vi "运维调试_采配水.vi"() -> ()   [LabVIEW 2016, in "PLC.lvlib"]
uses:
  PLC.lvlib
  <vilib>/Plasmionique/MB Master/MB_Master/MB_Master.lvclass
  <vilib>/Utility/miscctls.llb/LVPointTypeDef.ctl
  <vilib>/Plasmionique/MB Master/MB_Master_Serial/MB_Master_Serial.lvclass
  C:/Program Files (x86)/National Instruments/LabVIEW 2016/vi.lib/Plasmionique/MB Master/MB_Master/MB_Master.lvclass
  <vilib>/Instr/_visa.llb/VISA Configure Serial Port (Instr).vi
  <vilib>/Plasmionique/MB Master/MB Master.lvlib
panel:
  out "R118":i16 caption="多参数沉淀时间"
  in  "看门狗启用":bool
  out "R117":i16 caption="看门狗设置值"
  out "R33":i16 caption="看门狗计时器"
  in  "下载模式":bool
  in  "R116":i16(ring) caption="储水水体选择" items=["自来水", "采水泵"]
  out "当前启动泵号":u16(ring) items=["1号水样泵", "2号水样泵"]
  out "R113":i16 caption="储水时间设定"
  out "R25":i16
  in  "V14NC":bool
  out "R24":i16
  in  "V14NO":bool
  out "X2":bool caption="X1"
  out "采配水版本号":string
  out "R23":i16 caption="清洗频次计数"
  out "R112":i16 caption="清洗频次设定"
  out "R22":i16
  in  "V13NC":bool
  out "R111":i16 caption="排液时间"
  out "通讯故障":bool
  out "R21":i16
  in  "V13NO":bool
  out "R20":i16
  in  "M1-2":bool
  in  "潜水泵工作模式":u16(ring) items=["泵1单泵单管路", "泵2单泵单管路", "潜水泵双泵双管路", "自吸泵双泵双管路"]
  out "X11":bool caption="废液报警"
  out "X10":bool caption="自来水检测"
  out "X9":bool caption="泵2过载报警"
  out "X8":bool caption="泵1过载报警"
  out "X7":bool caption="断电检测"
  out "X6":bool caption="开门检测"
  out "X5":bool caption="烟雾检测"
  out "X4":bool caption="漏水检测"
  out "X3":bool caption="进样检测"
  out "X1":bool
  out "X0":bool caption="采样池液位开关"
  out "R109":i16 caption="配水时间"
  out "集成报警信息":string
  out "R108":i16 caption="自来水报警"
  out "R107":i16 caption="采水池液位报警设置"
  out "R106":i16 caption="进样超时设置"
  out "R105":i16 caption="二级清洗时间"
  out "R104":i16 caption="一级清洗时间"
  out "R103":i16 caption="外部管路清洗时间"
  out "R102":i16 caption="静置沉淀时间"
  out "R101":i16 caption="内部管路润洗时间"
  out "R100":i16 caption="外部管路润洗时间"
  out "R2":i16
  out "R1":i16
  out "多列列表框":i32(listbox)
  out "R19":i16
  in  "V6":bool
  out "R18":i16
  in  "V5":bool
  out "R17":i16
  in  "V4":bool
  out "R16":i16
  in  "V3":bool
  out "R15":i16
  in  "V2":bool
  out "R14":i16
  in  "M2":bool
  out "R13":i16
  in  "V1":bool
  out "R12":i16
  in  "M1-1":bool
  in  "返回":bool
  in  "参数设置":bool
  in  "单步启动":bool
  in  "启动":bool
  in  "停止":bool
  # "看门狗设置"
  # "S"
  # "S"
  # "S"
  # "S"
  # "次"
  # "次"
  # "S"
  # "S"
  # "S"
  # "S"
  # "S"
  # "S"
  # "S"
  # "S"
  # "S"
  # "S"
  # "S"
  # "单步计时："
  # "s"
  # "流程计时："
  # "s"
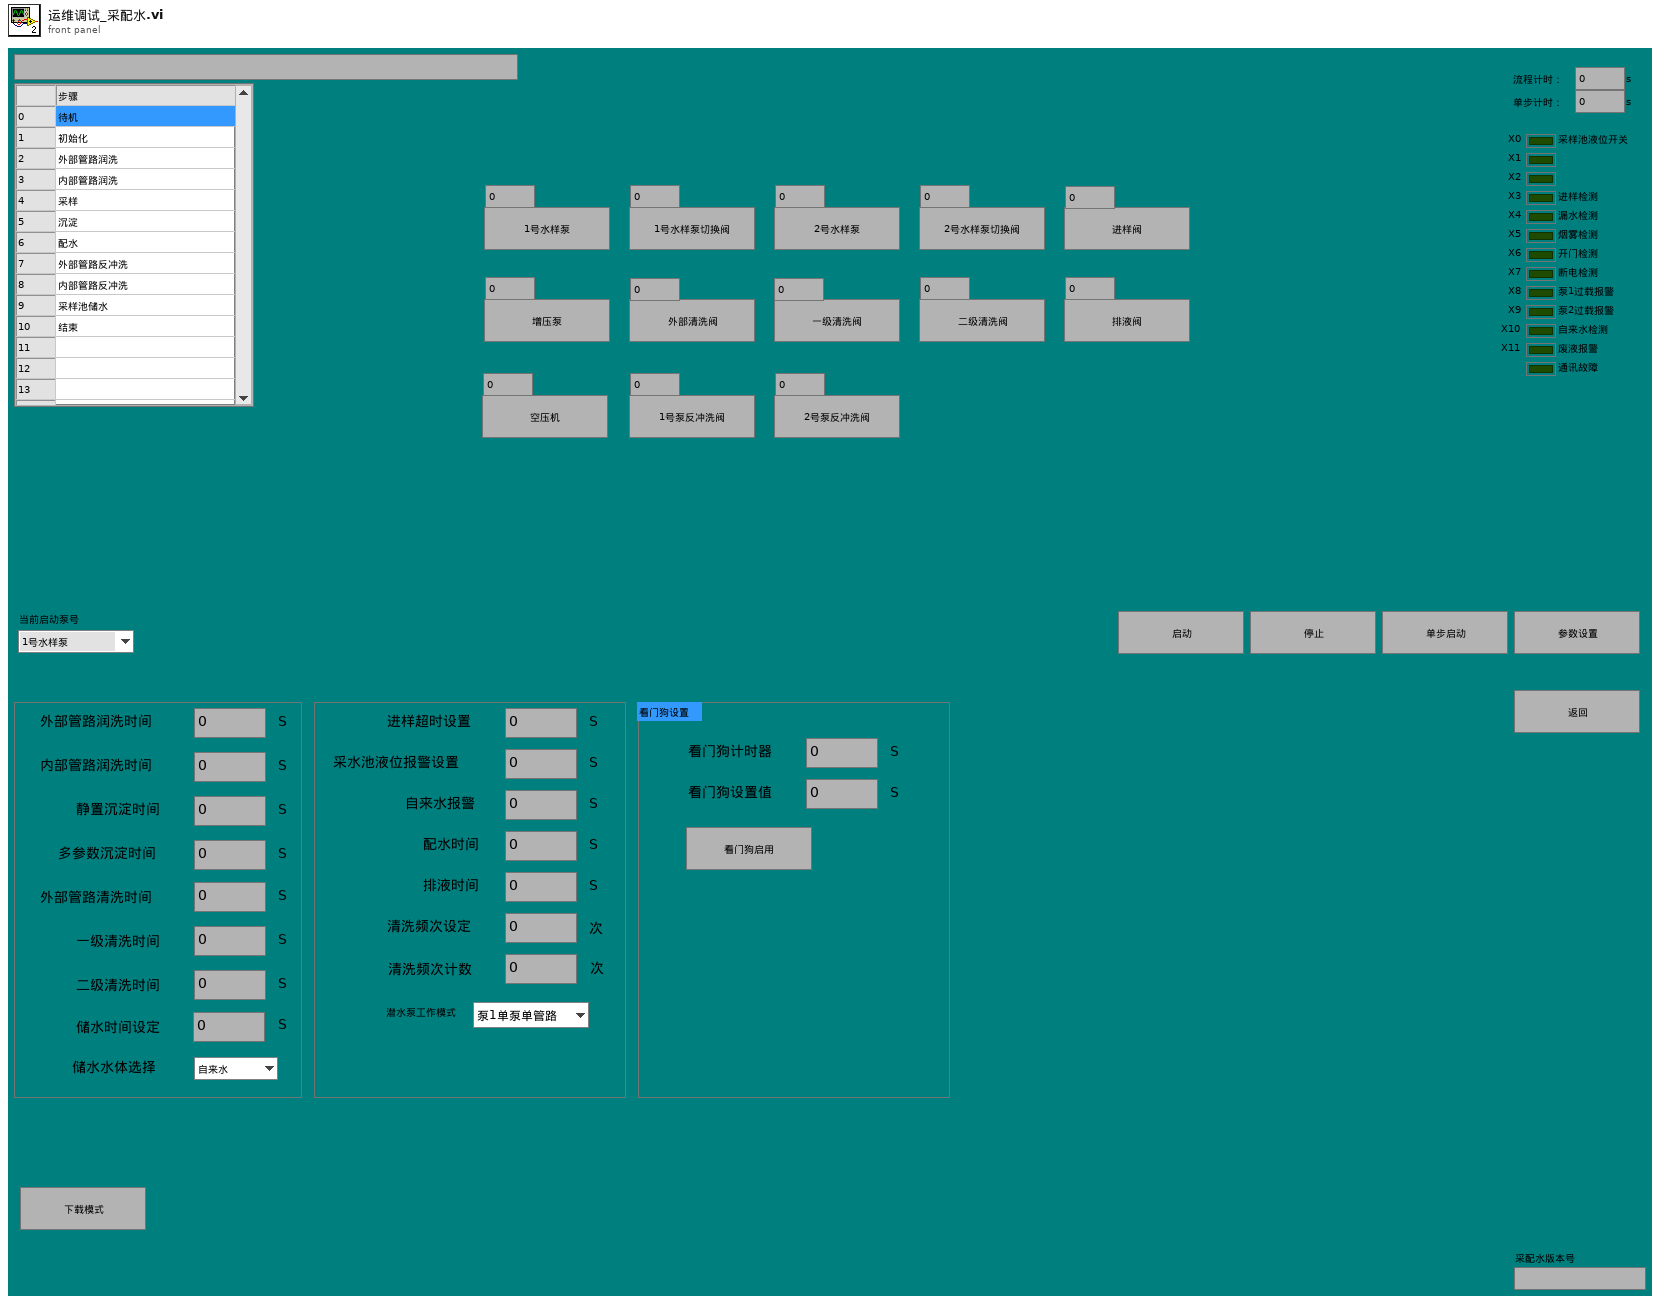
[diagram p1: front panel]
types:
  T1 = typedef "LVPointTypeDef.ctl" = cluster{"Horizontal":i16, "Vertical":i16}
  T2 = cluster{"命令":string, "数据":cluster{"starting address":u16, "holding register value":u16}}
  T3 = cluster{"时间标识":timestamp, "设备":string, "日志信息":string}
  T4 = cluster{"R0":i16, "R1":i16, "R2":i16, "R3":i16, "R4":i16, "R5":i16, "R6":i16, "R7":i16, "R8":i16, "R9":i16, "R10":i16, "R11":i16, "R12":i16, "R13":i16, "R14":i16, "R15":i16, "R16":i16, "R17":i16, "R18":i16, "R19":i16, "R20":i16, "R21":i16, "R22":i16, "R23":i16, "R24":i16, "R25":i16, "R26":i16, "R27":i16, "R28":i16, "R29":i16, "R30":i16, "R31":i16, "R32":i16, "R33":i16, "R34":i16}
  T5 = cluster{"R100":i16, "R101":i16, "R102":i16, "R103":i16, "R104":i16, "R105":i16, "R106":i16, "R107":i16, "R108":i16, "R109":i16, "R110":i16, "R111":i16, "R112":i16, "R113":i16, "R114":i16, "R115":i16, "R116":i16, "R117":i16, "R118":i16, "R119":i16}
  T6 = cluster{"seconds since 1Jan1904":timestamp, "table输入":string, string, "table输入":string}
  T7 = cluster{"时间标识":timestamp, "设备":string, "日志信息":string, "流程参数":string}
  T8 = cluster{"命令":string, cluster{"starting address":u16, "holding register value":u16}}
  T9 = cluster{"命令":string, "数据":cluster{"starting address":u16, "holding register values":u16[]}}
  T10 = cluster{"命令":string, "data":cluster{"starting address":u16, "coil values":bool[]}}
  T11 = cluster{"测试模式":enum16{"正常测试", "集成干预"}, "参数启用":cluster{"氨氮":bool, "总磷总氮":bool, "CODMn":bool, "CODcr":bool, "多参数":bool}}
  T12 = enum32{"Bad", "Idle", "Run top level", "Running"}
  T13 = cluster{"baud rate (bps)":u32, "stop bits":u16, "parity":u16, "flow control":u16, "timeout":u32, "retries":i32}
  T14 = cluster{"starting address":u16, "holding register values":u16[]}
  T15 = cluster{"starting address":u16, "holding register value":u16}
  T16 = cluster{"starting address":u16, "coil values":bool[]}
  T17 = cluster{"Registers[0]":u16, "Registers[1]":u16, "Registers[2]":u16, "Registers[3]":u16, "Registers[4]":u16, "Registers[5]":u16, "Registers[6]":u16, "Registers[7]":u16, "Registers[8]":u16, "Registers[9]":u16, "Registers[10]":u16, "Registers[11]":u16, "Registers[12]":u16, "Registers[13]":u16, "Registers[14]":u16, "Registers[15]":u16, "Registers[16]":u16, "Registers[17]":u16, "Registers[18]":u16, "Registers[19]":u16, "Registers[20]":u16, "Registers[21]":u16, "Registers[22]":u16, "Registers[23]":u16, "Registers[24]":u16, "Registers[25]":u16, "Registers[26]":u16, "Registers[27]":u16, "Registers[28]":u16, "Registers[29]":u16, "Registers[30]":u16, "Registers[31]":u16, "Registers[32]":u16, "Registers[33]":u16, "Registers[34]":u16}
  T18 = cluster{"数组 2[0]":sgl, "数组 2[1]":sgl, "数组 2[2]":sgl, "数组 2[3]":sgl, "数组 2[4]":sgl}
  T19 = cluster{"Registers[0]":u16, "Registers[1]":u16, "Registers[2]":u16, "Registers[3]":u16, "Registers[4]":u16, "Registers[5]":u16}
  T20 = cluster{"Registers[0]":u16, "Registers[1]":u16, "Registers[2]":u16, "Registers[3]":u16, "Registers[4]":u16, "Registers[5]":u16, "Registers[6]":u16, "Registers[7]":u16, "Registers[8]":u16, "Registers[9]":u16, "Registers[10]":u16, "Registers[11]":u16, "Registers[12]":u16, "Registers[13]":u16, "Registers[14]":u16, "Registers[15]":u16, "Registers[16]":u16, "Registers[17]":u16, "Registers[18]":u16, "Registers[19]":u16}
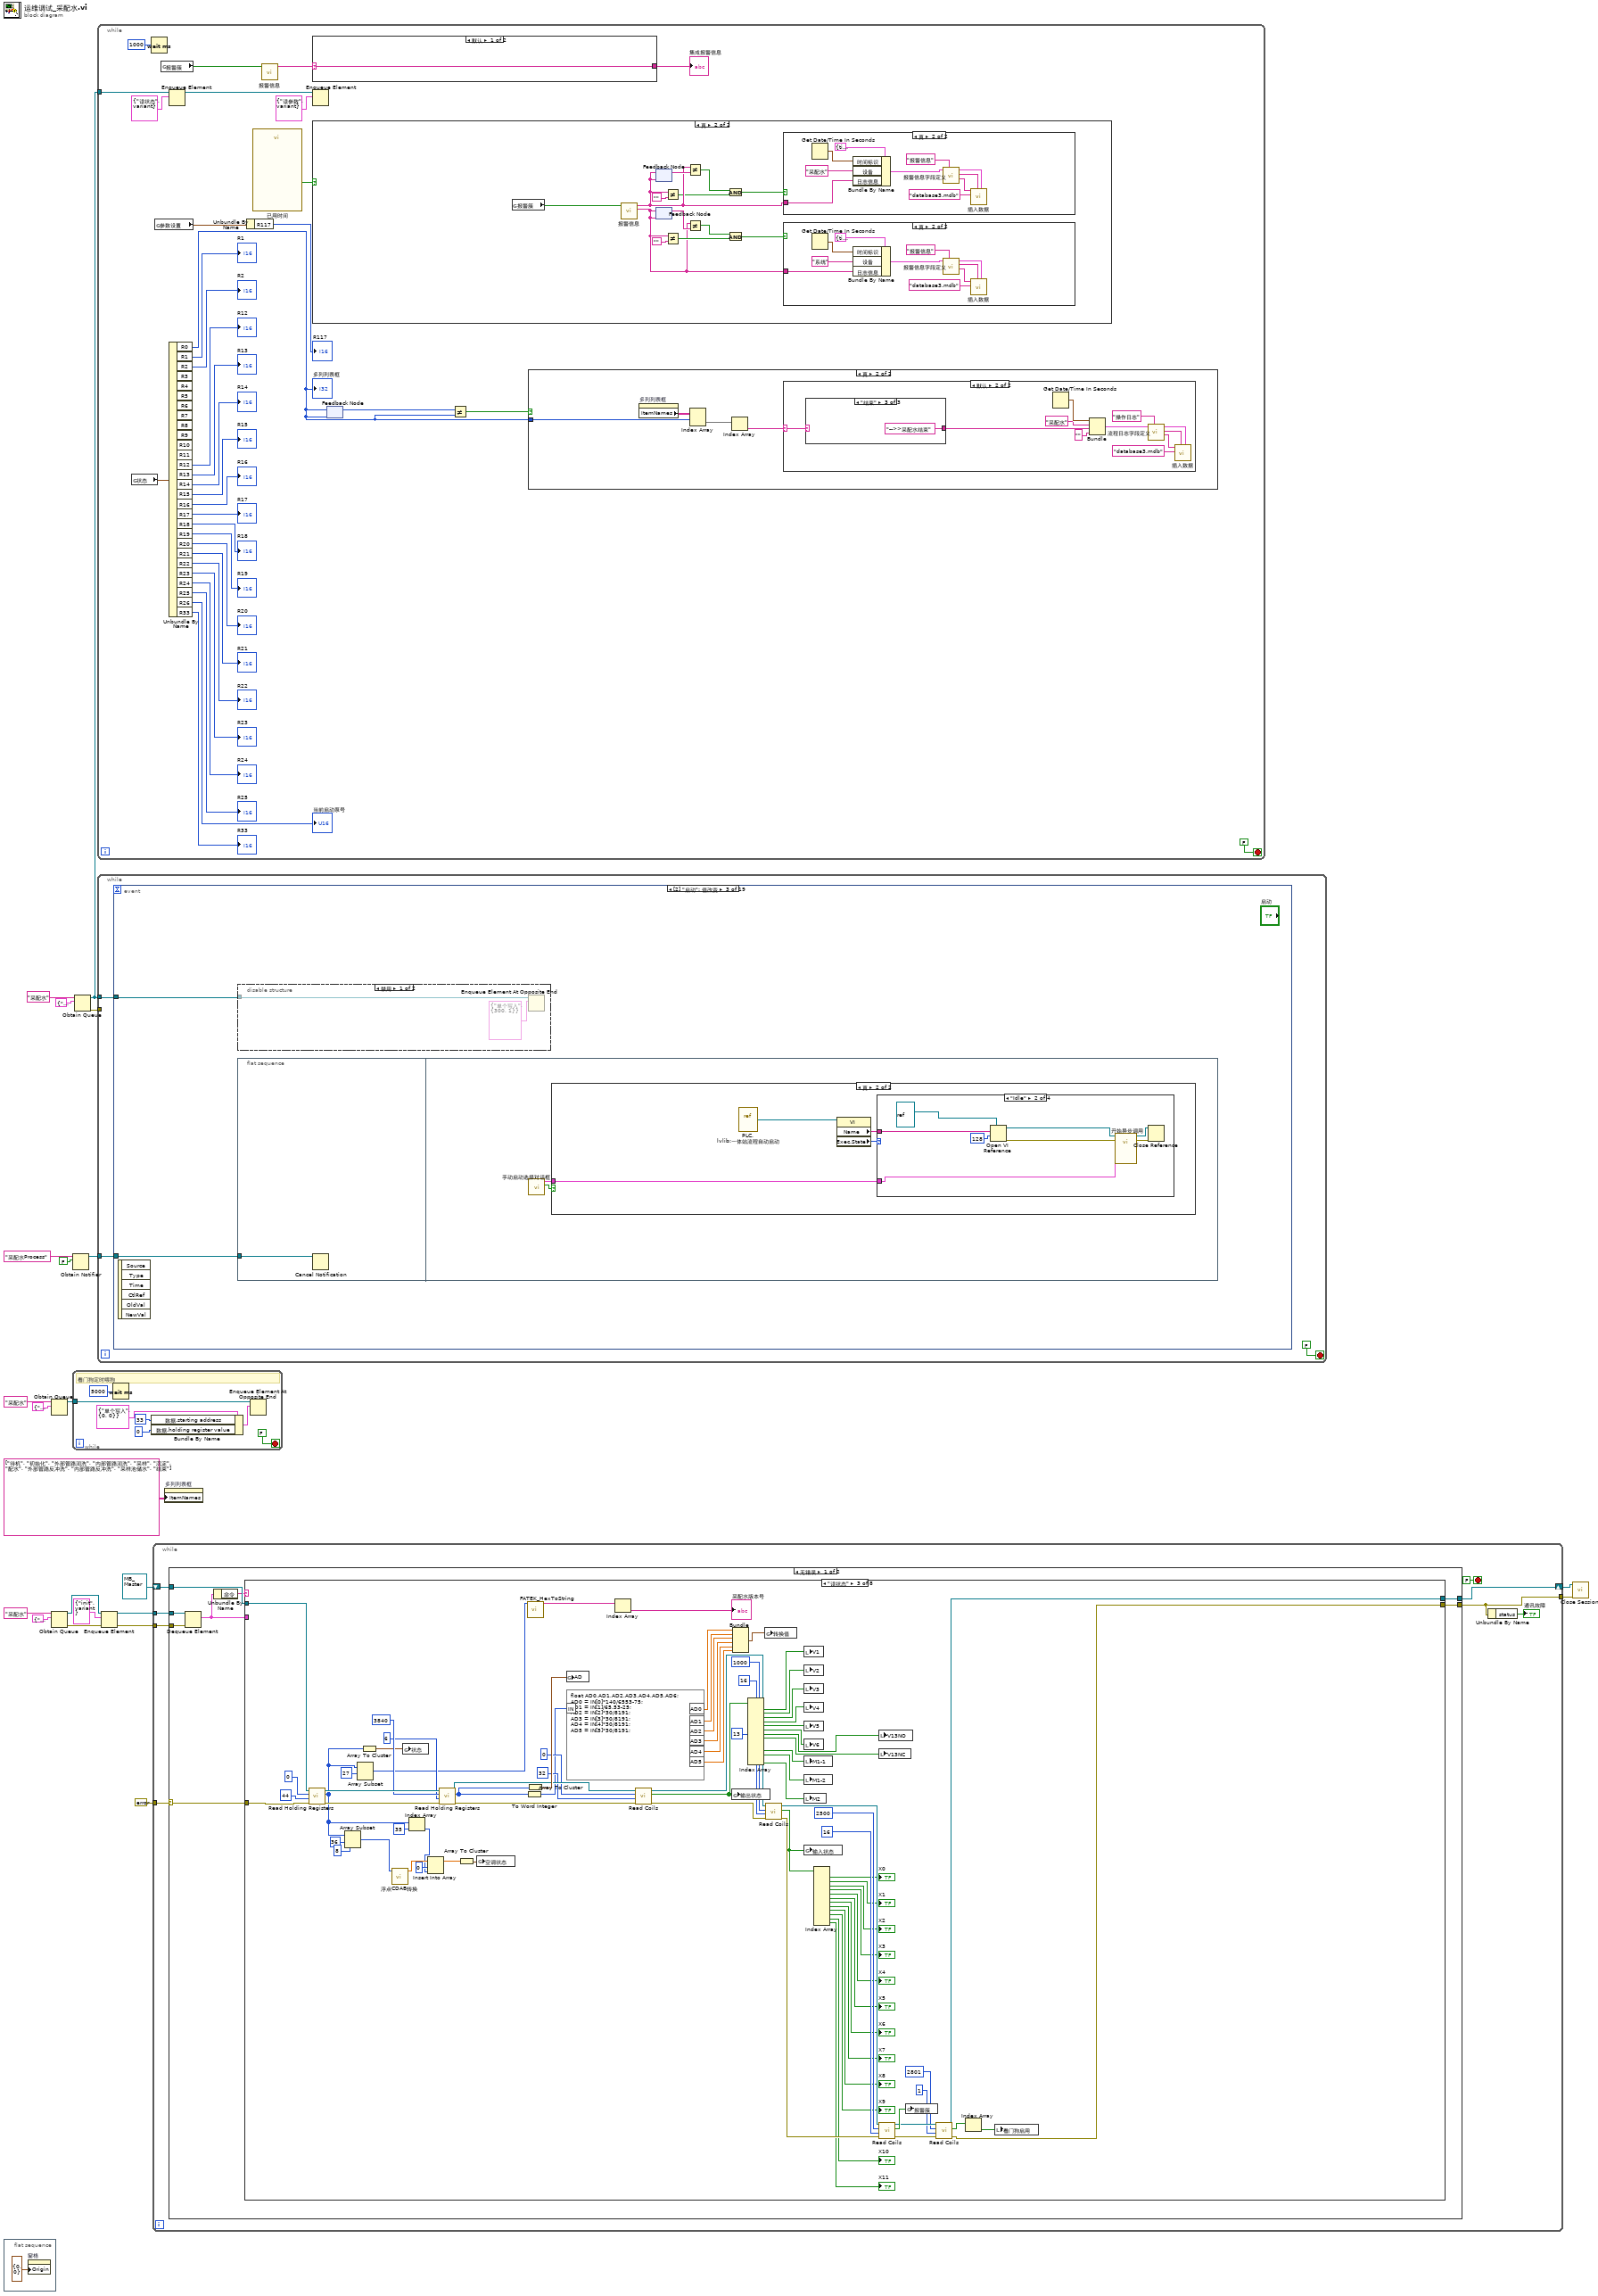
[diagram p0: block diagram]
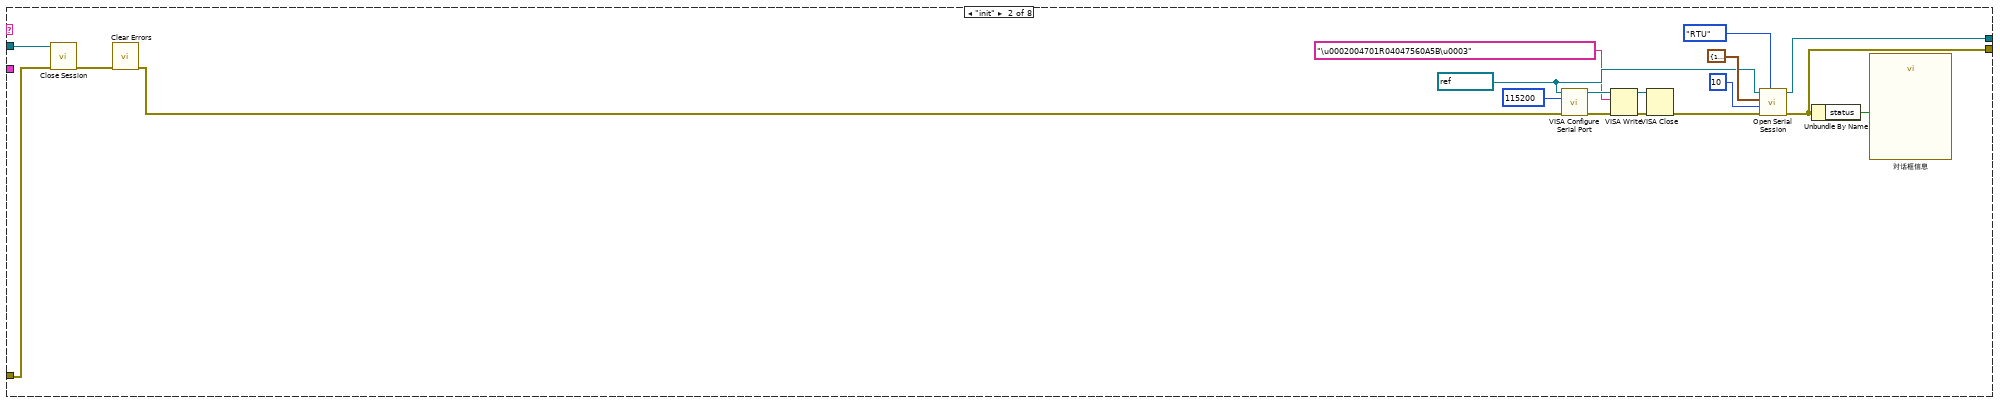
[diagram p3: hidden frame]
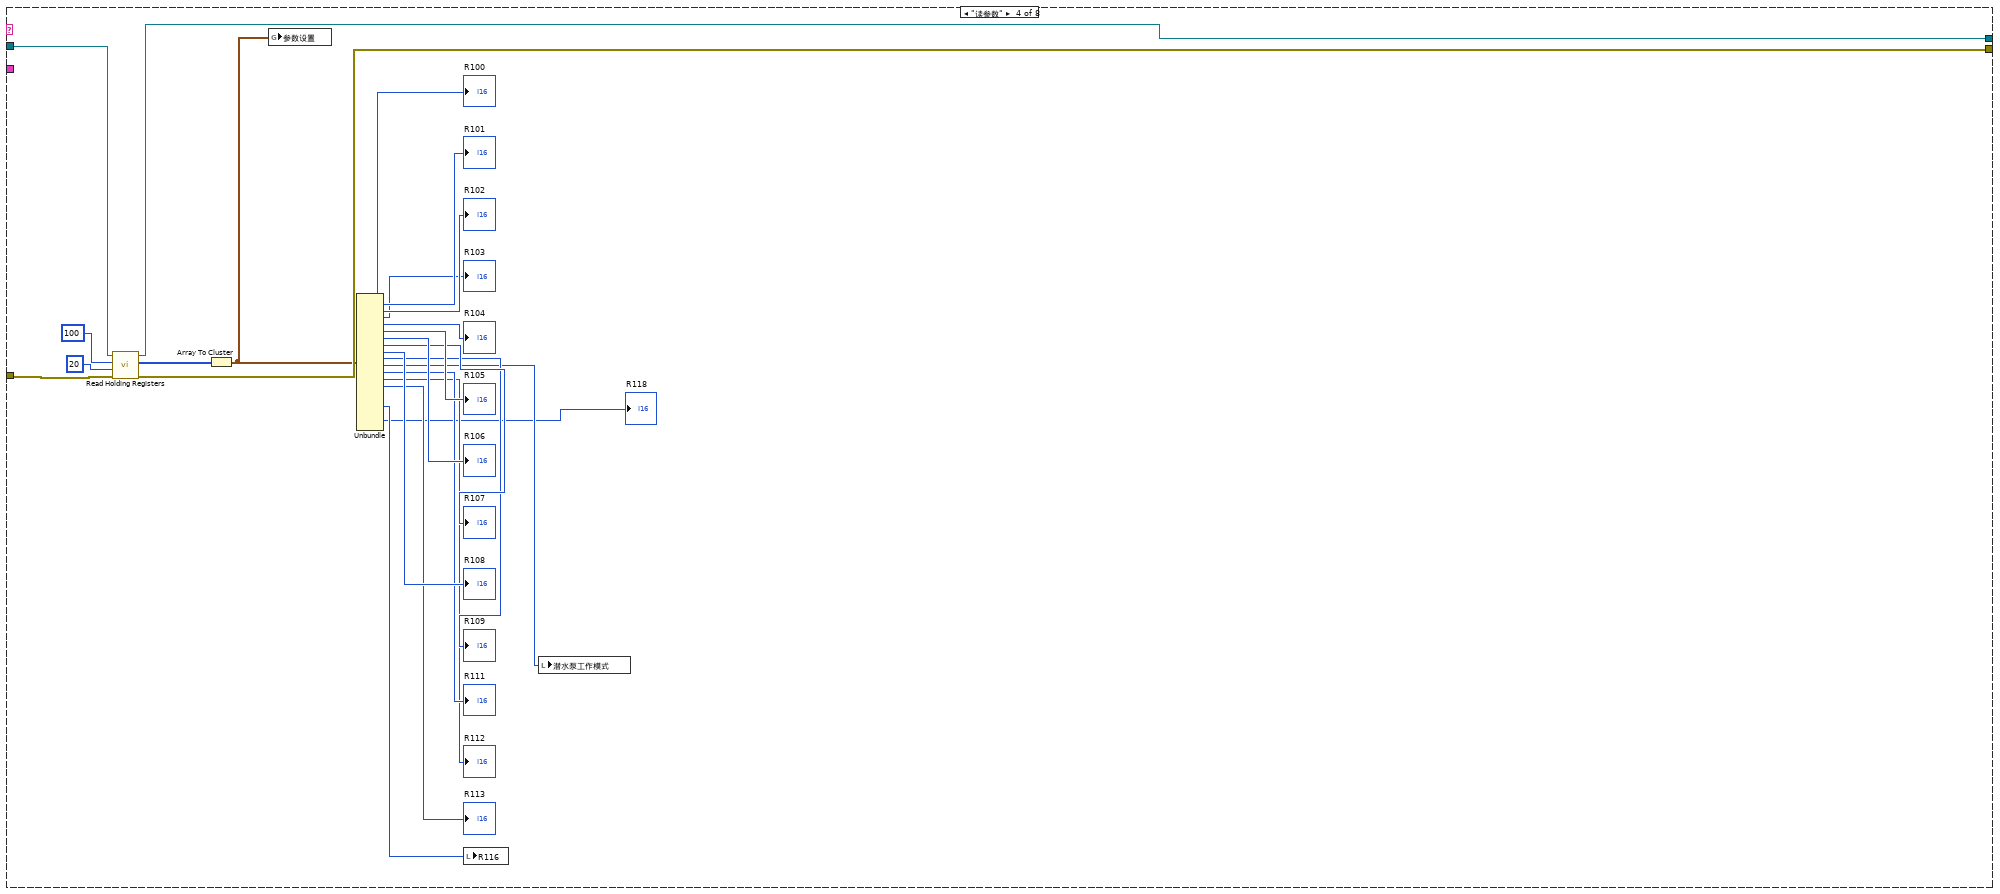
[diagram p4: hidden frame]
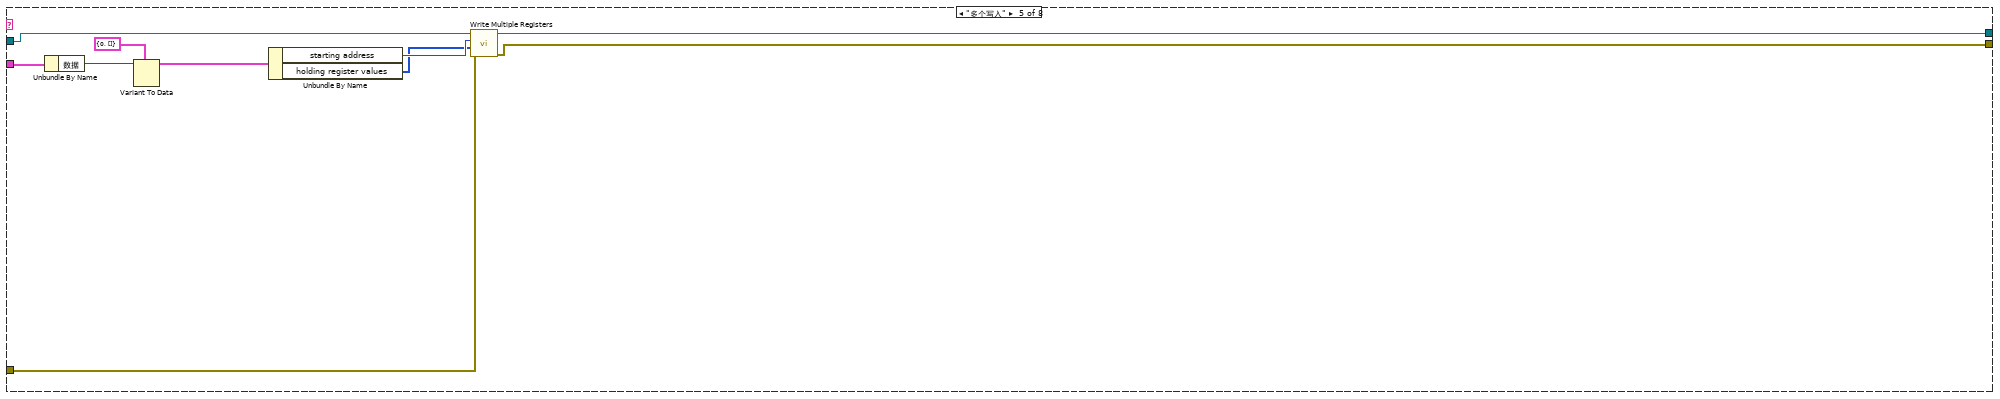
[diagram p5: hidden frame]
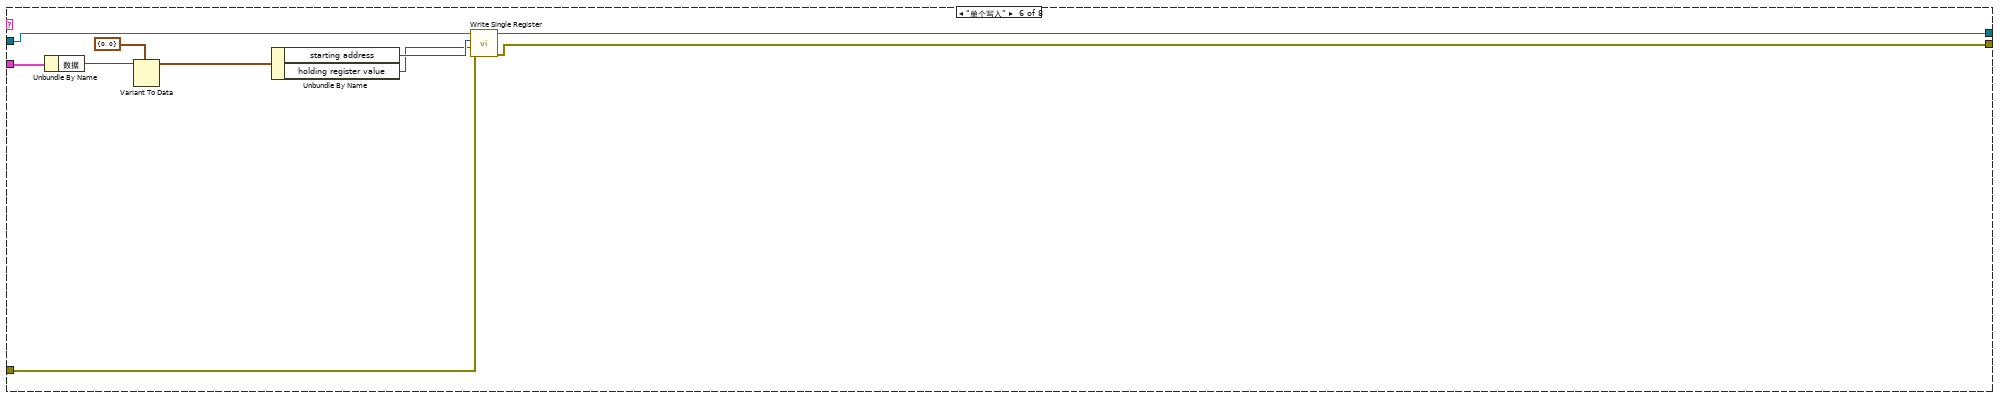
[diagram p6: hidden frame]
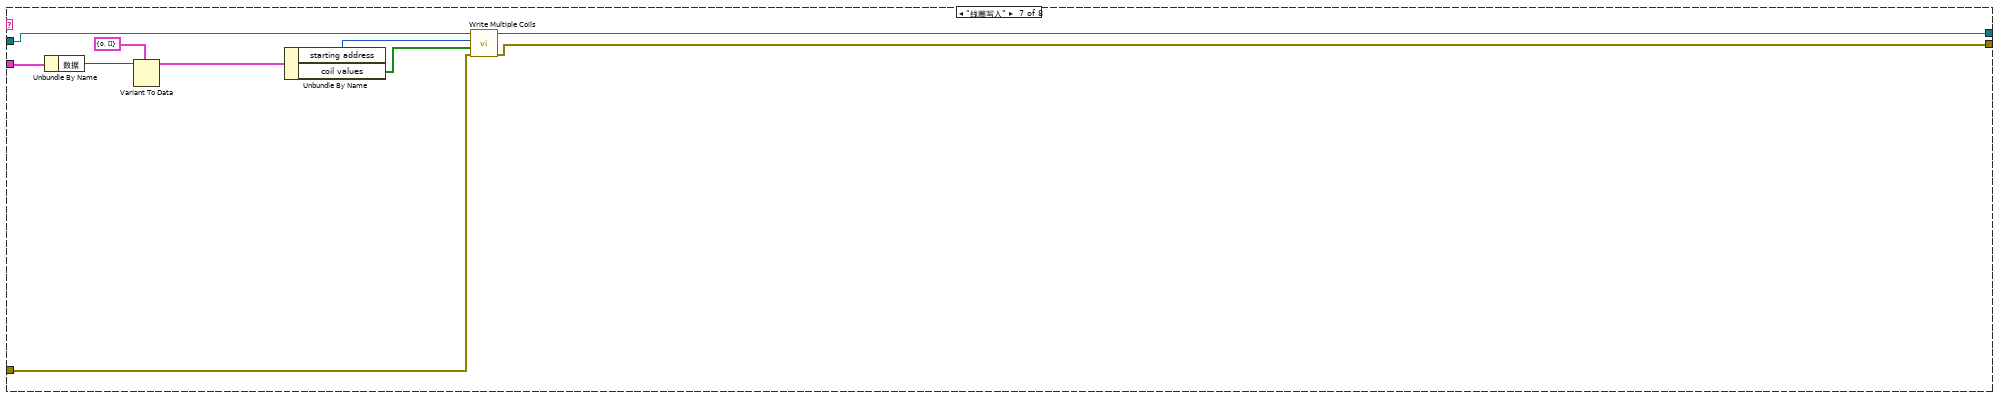
[diagram p7: hidden frame]
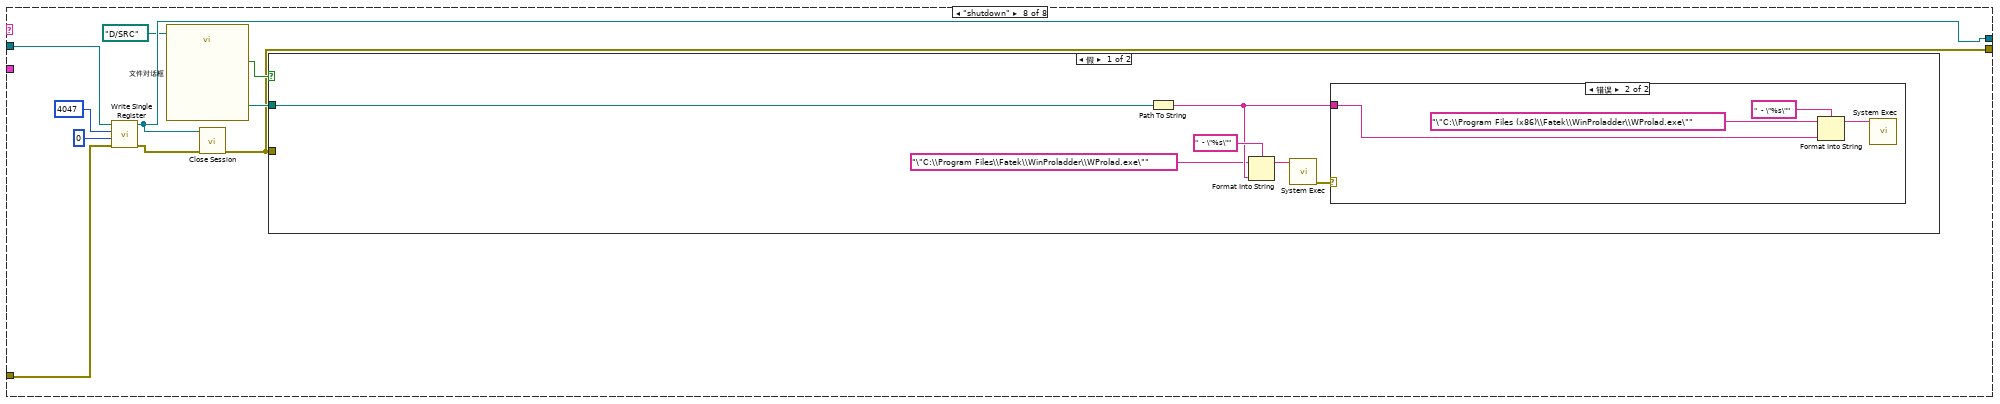
[diagram p8: hidden frame]
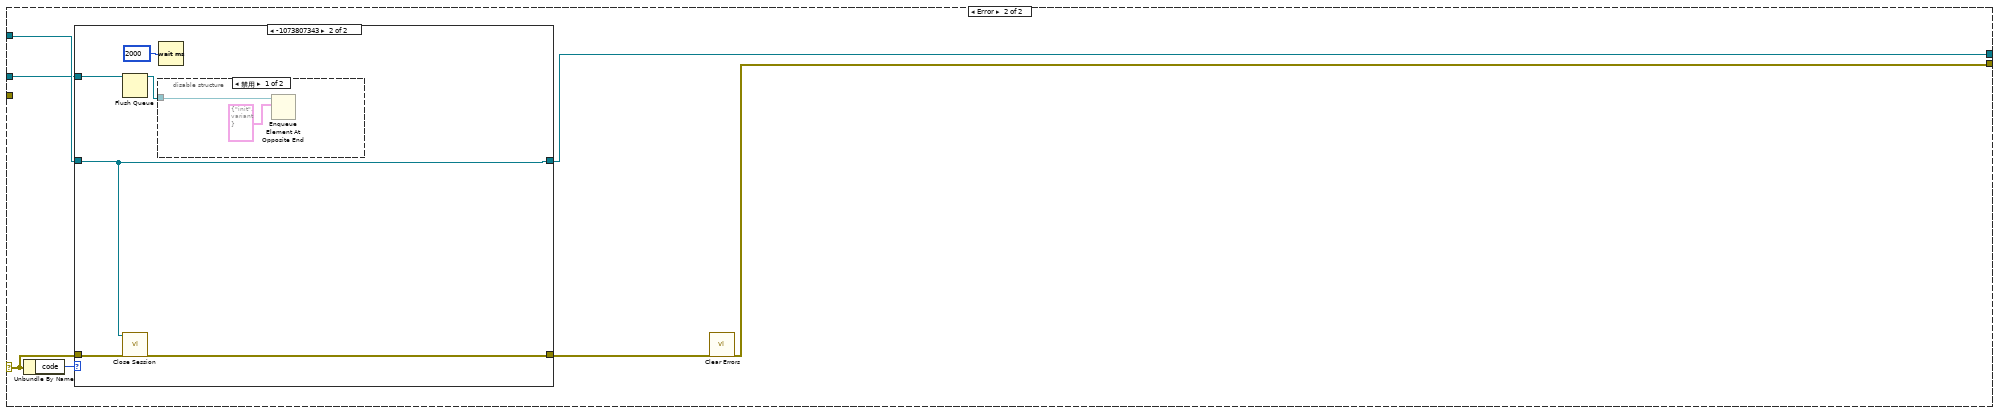
[diagram p11: hidden frame]
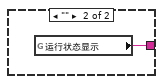
[diagram p17: hidden frame]
diagram:
  n1 = flat-sequence {
    frame #0 {
      n2 = property on="窗格" class="Pane"("Origin"=T1 {"Horizontal"=0, "Vertical"=0} ("原点")) -> ()  [unwired: 2 in, 2 out]
    }
  }
  n3 = Obtain Queue(name (unnamed)="采配水" ("名称（未命名）"), element data type=cluster{"命令":string, "数据":variant} {"命令"="", "数据"=variant}) -> (queue out=w1:refnum<queue>)  [unwired: 3 in, 2 out]
  n4 = Obtain Queue(name (unnamed)="采配水" ("名称（未命名）"), element data type=cluster{"命令":string, "数据":variant} {"命令"="", "数据"=variant}) -> (queue out=w12:refnum<queue>, error out=w11:errorcluster)  [unwired: 3 in, 1 out]
  n5 = Obtain Notifier(name (unnamed)="采配水Process" ("名称（未命名）"), notification data type=FALSE) -> (notifier out=w15:refnum<notifier>)  [unwired: 2 in, 2 out]
  n6 = while {
    tunnel: w1 -> [w26]
    stop <- FALSE stop-if-true
    # "看门狗定时喂狗"
    n7 = Wait (ms)(milliseconds to wait=u32 5000 ("等待时间（毫秒）")) -> ()  [unwired: 1 out]
    n8 = Bundle By Name(cluster=T2 {"命令"="单个写入", "数据"={"starting address"=0, "holding register value"=0}} ("元素"), "数据.starting address"=u16 33, "数据.holding register value"=u16 0) -> (w27:T2)
    n9 = Enqueue Element At Opposite End(queue=w26, element=w27) -> ()  [unwired: 2 in, 3 out]
  }
  n10 = Obtain Queue(name (unnamed)="采配水" ("名称（未命名）"), element data type=cluster{"命令":string, "数据":variant} {"命令"="", "数据"=variant}) -> (queue out=w19:refnum<queue>, error out=w20:errorcluster)  [unwired: 3 in, 1 out]
  n11 = while {
    tunnel: w19 -> [w63]
    stop <- FALSE stop-if-true
    n12 = global read "采配水全局变量.vi" "状态"() -> (w61:T4)
    n13 = Wait (ms)(milliseconds to wait=u32 1000 ("等待时间（毫秒）")) -> ()  [unwired: 1 out]
    n14 = global read "采配水全局变量.vi" "参数设置"() -> (w32:T5)
    n15 = global read "采配水全局变量.vi" "报警簇"() -> (w49:bool[])
    n16 = Enqueue Element(queue=w63, element=cluster{"命令":string, "数据":variant} {"命令"="读状态", "数据"=variant} ("元素")) -> (queue out=w44:refnum<queue>)  [unwired: 2 in, 2 out]
    n17 = Unbundle By Name(w61) -> ("R0"=w42:i16, "R1"=→"R1":i16, "R2"=→"R2":i16, "R12"=→"R12":i16, "R13"=→"R13":i16, "R14"=→"R14":i16, "R15"=→"R15":i16, "R16"=→"R16":i16, "R17"=→"R17":i16, "R18"=→"R18":i16, "R19"=→"R19":i16, "R20"=→"R20":i16, "R21"=→"R21":i16, "R22"=→"R22":i16, "R23"=→"R23":i16, "R24"=→"R24":i16, "R25"=→"R25":i16, "R26"=→"当前启动泵号":i16, "R33"=→"R33":i16)  [unwired: 9 out]
    "多列列表框" <- w42
    n18 = Unbundle By Name(w32) -> ("R117"=→"R117":i16)
    n19 = call "已用时间"() -> ("Time has Elapsed"=w47:bool)  [unwired: 12 in, 7 out]
    n20 = call "报警信息.vi"("报警簇"=w49) -> ("采配水报警信息"=w41:string)  [unwired: 9 in, 1 out]
    n21 = case shown="默认" w41 {
      selector: w41 -> [w98 _]
      tunnel: [w98 w99] -> w48
      frame Default {
      }
      frame "" {
        n22 = global read "采配水全局变量.vi" "运行状态显示"() -> (w99:string)
      }
    }
    "集成报警信息" <- w48
    n23 = Enqueue Element(queue=w44, element=cluster{"命令":string, "数据":variant} {"命令"="读参数", "数据"=variant} ("元素")) -> ()  [unwired: 2 in, 3 out]
    n24 = case shown="真" w47 {
      frame False {
      }
      frame True {
        n25 = global read "采配水全局变量.vi" "报警簇"() -> (w77:bool[])
        n26 = call "报警信息.vi"("报警簇"=w77) -> ("系统报警信息"=w66:string, "采配水报警信息"=w73:string)  [unwired: 9 in]
        n27 = feedback #1(w73) -> (w76:string)
        n28 = feedback-in #1(w73) -> ()
        n29 = feedback #2(w66) -> (w67:string)
        n30 = feedback-in #2(w66) -> ()
        n31 = Not Equal?(x=w73, y="") -> (x != y?=w71:bool)
        n32 = Not Equal?(x=w66, y="") -> (x != y?=w70:bool)
        n33 = Not Equal?(x=w73, y=w76) -> (x != y?=w75:bool)
        n34 = Not Equal?(x=w66, y=w67) -> (x != y?=w68:bool)
        n35 = And(x=w75, y=w71) -> (x .and. y?=w74:bool)
        n36 = And(x=w68, y=w70) -> (x .and. y?=w65:bool)
        n37 = case shown="真" w74 {
          tunnel: w73 -> [_ w88]
          frame False {
          }
          frame True {
            n38 = Get Date/Time In Seconds() -> (seconds since 1Jan1904=w90:timestamp)
            n39 = Bundle By Name(cluster=T3 {"时间标识"=timestamp(0 s since 1904-01-01), "设备"="", "日志信息"=""} ("data in"), "时间标识"=w90, "设备"="采配水", "日志信息"=w88) -> (w91:T3)
            n40 = call "报警信息字段定义.vi"("table输入"="报警信息", "data in"=w91) -> ("table输出"=w95:string, "columns"=w96:string[], "data out"=w97:T3)  [unwired: 7 in]
            n41 = call "插入数据.vi"("data"=w97, "columns"=w96, "database"="database3.mdb", "table"=w95) -> ()  [unwired: 7 in, 1 out]
          }
        }
        n42 = case shown="真" w65 {
          tunnel: w66 -> [_ w78]
          frame False {
          }
          frame True {
            n43 = Get Date/Time In Seconds() -> (seconds since 1Jan1904=w80:timestamp)
            n44 = Bundle By Name(cluster=T3 {"时间标识"=timestamp(0 s since 1904-01-01), "设备"="", "日志信息"=""} ("data in"), "时间标识"=w80, "设备"="系统", "日志信息"=w78) -> (w81:T3)
            n45 = call "报警信息字段定义.vi"("table输入"="报警信息", "data in"=w81) -> ("table输出"=w85:string, "columns"=w86:string[], "data out"=w87:T3)  [unwired: 7 in]
            n46 = call "插入数据.vi"("data"=w87, "columns"=w86, "database"="database3.mdb", "table"=w85) -> ()  [unwired: 7 in, 1 out]
          }
        }
      }
    }
    n47 = feedback-in #3(w42) -> ()
    n48 = feedback #3(w42) -> (w43:i16)
    n49 = Not Equal?(x=w43, y=w42) -> (x != y?=w50:bool)
    n50 = case shown="真" w50 {
      tunnel: w42 -> [_ w102]
      frame False {
      }
      frame True {
        n51 = property on="多列列表框" class="MCListbox (严格)"() -> ("ItemNames"=w103:string[][])  [unwired: 2 in, 2 out]
        n52 = Index Array(array=w103, index (row)=w102) -> (element=w101:string[])  [unwired: 1 in]
        n53 = Index Array(array=w101) -> (element=w100:string)  [unwired: 1 in]
        n54 = case shown="默认" w100 {
          selector: w100 -> [_ w105]
          frame "待机" {
          }
          frame Default {
            n55 = case shown="\"结束\"" w105 {
              selector: w105 -> [w115 _ _]
              tunnel: [w115 "-->>采配水初始化" "-->>采配水结束"] -> w104
              frame Default {
              }
              frame "初始化" {
              }
              frame "结束" {
              }
            }
            n56 = Get Date/Time In Seconds() -> (seconds since 1Jan1904=w109:timestamp)
            n57 = Bundle("seconds since 1Jan1904"=w109, "table输入"="采配水", w104, "table输入"="") -> (w107:T6)  [unwired: 1 in]
            n58 = call "流程日志字段定义.vi"("table输入"="操作日志", "data in"=w107) -> ("table输出"=w112:string, "columns"=w113:string[], "data out"=w114:T7)  [unwired: 7 in]
            n59 = call "插入数据.vi"("data"=w114, "columns"=w113, "database"="database3.mdb", "table"=w112) -> ()  [unwired: 7 in, 1 out]
          }
        }
      }
    }
  }
  n60 = while {
    tunnel: w19 -> [w119]
    tunnel: w20 -> [_]
    tunnel: w15 -> [w118]
    stop <- FALSE stop-if-true
    n61 = event shown="[2] \"启动\": 值改变" {
      selector: _ -> [_ _ _ _ _ _ _ _ _ _ _ _ _ _ _ _ _ _ _]
      dyn-events: _ -> [_ _ _ _ _ _ _ _ _ _ _ _ _ _ _ _ _ _ _]
      timeout: _ -> [_ _ _ _ _ _ _ _ _ _ _ _ _ _ _ _ _ _ _]
      tunnel: w119 -> [_ w123 w126 w148 w167 w172 w178 w189 _ _ _ _ w217 w219 w224 w229 w234 w239 w244]
      tunnel: w118 -> [_ w122 w125 _ _ _ _ _ _ _ _ _ _ _ _ _ _ _ _]
      event Timeout {
        n62 = event-data() -> ()  [unwired: 1 in, 3 out]
      }
      event "停止": Value Change {
        n63 = event-data() -> ()  [unwired: 1 in, 6 out]
        n64 = Send Notification(notification=TRUE ("通知"), notifier=w122) -> ()  [unwired: 1 in, 2 out]
        n65 = Enqueue Element At Opposite End(queue=w123, element=T8 {"命令"="单个写入", {"starting address"=300, "holding register value"=2}} ("元素")) -> ()  [unwired: 2 in, 3 out]
      }
      event "启动": Value Change {
        n66 = event-data() -> ()  [unwired: 1 in, 6 out]
        n67 = disable-structure shown="禁用" {
          disable-tunnel: w126 -> [w144 _]
          frame Disabled {
            n68 = Enqueue Element At Opposite End(queue=w144, element=T8 {"命令"="单个写入", {"starting address"=300, "holding register value"=1}} ("元素")) -> ()  [unwired: 2 in, 3 out]
          }
          frame Enabled {
          }
        }
        n69 = flat-sequence {
          tunnel: w125 -> [w127]
          frame #0 {
            n70 = Cancel Notification(0:w127) -> ()  [unwired: 1 in, 3 out]
          }
          frame #1 {
            n71 = call "手动启动选择对话框.vi"() -> ("确定"=w129:bool, "参数"=w128:T11)  [unwired: 10 in]
            n72 = case shown="真" w129 {
              tunnel: w128 -> [_ w130]
              frame False {
              }
              frame True {
                n73 = vi-ref "PLC.lvlib:一体站流程自动启动.vi"() -> (w133:refnum<vi>)
                n74 = property class="VI"(reference=w133) -> ("Name"=w132:string, "Exec.State"=w131:T12)  [unwired: 1 in, 2 out]
                n75 = case shown="\"Idle\"" w131 {
                  tunnel: w132 -> [_ w141 _ _]
                  tunnel: w130 -> [_ w135 _ _]
                  frame "Bad", Default {
                  }
                  frame "Idle" {
                    n76 = Open VI Reference(type specifier VI Refnum (for type only)=refnum<vi> refnum, vi path=w141, options=128 ("选项")) -> (vi reference=w139:refnum<vi>, error out=w137:errorcluster)  [unwired: 3 in]
                    n77 = call-by-ref "开始异步调用"(reference=w139, error in=w137, "参数"=w135) -> (reference out=w138:refnum<vi>, error out=w136:errorcluster)  [unwired: 11 in]
                    n78 = Close Reference(reference=w138, error in (no error)=w136) -> ()  [unwired: 1 out]
                  }
                  frame "Run top level" {
                  }
                  frame "Running" {
                    n79 = One Button Dialog(message="流程已经运行,无须重复启动" ("消息")) -> ()  [unwired: 1 in, 1 out]
                  }
                }
              }
            }
          }
        }
      }
      event "单步启动": Value Change {
        n80 = event-data() -> ()  [unwired: 1 in, 6 out]
        n81 = call "单步启动对话框.vi"() -> ("单步启动步骤输出"=w145:u16)  [unwired: 11 in]
        n82 = Bundle By Name(cluster=T2 {"命令"="单个写入", "数据"={"starting address"=301, "holding register value"=0}} ("元素"), "数据.holding register value"=w145) -> (w146:T2)
        n83 = Enqueue Element At Opposite End(queue=w148, element=w146) -> ()  [unwired: 2 in, 3 out]
      }
      event "R100", "R101", "R102", "R103", "R104", "R105", "R106", "R107", "R108", "R109", "潜水泵工作模式", "R111", "R112", "R113": Value Change {
        n84 = event-data() -> ()  [unwired: 1 in, 6 out]
        n85 = local read "R100"() -> (w162:i16)
        n86 = local read "R101"() -> (w161:i16)
        n87 = local read "R102"() -> (w160:i16)
        n88 = local read "R103"() -> (w159:i16)
        n89 = local read "R104"() -> (w158:i16)
        n90 = local read "R105"() -> (w157:i16)
        n91 = local read "R106"() -> (w156:i16)
        n92 = local read "R107"() -> (w155:i16)
        n93 = local read "R108"() -> (w154:i16)
        n94 = local read "R109"() -> (w153:i16)
        n95 = local read "R111"() -> (w151:i16)
        n96 = local read "R112"() -> (w150:i16)
        n97 = local read "R113"() -> (w149:i16)
        n98 = Build Array(w162, w161, w160, w159, w158, w157, w156, w155, w154, w153, "潜水泵工作模式", w151, w150, w149) -> (w163:u16[])
        n99 = Bundle By Name(cluster=T9 {"命令"="多个写入", "数据"={"starting address"=0, "holding register values"=[]}} ("元素"), "数据.starting address"=u16 100, "数据.holding register values"=w163) -> (w164:T9)
        n100 = Enqueue Element At Opposite End(queue=w167, element=w164) -> ()  [unwired: 2 in, 3 out]
      }
      event "R116", "R117", "R118": Value Change {
        n101 = event-data() -> ()  [unwired: 1 in, 6 out]
        n102 = local read "R117"() -> (w169:i16)
        n103 = local read "R118"() -> (w168:i16)
        n104 = Build Array("R116", w169, w168) -> (w171:i16[])
        n105 = Bundle By Name(cluster=T9 {"命令"="多个写入", "数据"={"starting address"=0, "holding register values"=[]}} ("元素"), "数据.starting address"=u16 116, "数据.holding register values"=w171) -> (w173:T9)
        n106 = Enqueue Element At Opposite End(queue=w172, element=w173) -> ()  [unwired: 2 in, 3 out]
      }
      event "下载模式": Value Change {
        n107 = event-data() -> ("NewVal"=w177:bool)  [unwired: 1 in, 5 out]
        n108 = Flush Queue(queue=w178) -> (queue out=w176:refnum<queue>)  [unwired: 1 in, 2 out]
        n109 = case shown="真" w177 {
          tunnel: w176 -> [w179 w183]
          frame False {
            n110 = Enqueue Element At Opposite End(queue=w179, element=cluster{"命令":string, "数据":variant} {"命令"="init", "数据"=variant} ("元素")) -> ()  [unwired: 2 in, 3 out]
          }
          frame True {
            n111 = Two Button Dialog(message="请再次确认是否切换为下载模式，切换为下载模式将导致采配水工作异常，非专业人员请勿进行此操作！" ("消息")) -> (T button?=w181:bool)  [unwired: 2 in]
            n112 = case shown="真" w181 {
              tunnel: w183 -> [_ w186]
              frame False {
                n113 = local write "下载模式"(FALSE ("下载模式")) -> ()
              }
              frame True {
                n114 = Enqueue Element At Opposite End(queue=w186, element=cluster{"命令":string, "数据":variant} {"命令"="shutdown", "数据"=variant} ("元素")) -> ()  [unwired: 2 in, 3 out]
              }
            }
          }
        }
      }
      event "R23": Value Change {
        n115 = event-data() -> ()  [unwired: 1 in, 6 out]
        n116 = local read "R23"() -> (w188:i16)
        n117 = Build Array(w188) -> (w187:i16[])
        n118 = Bundle By Name(cluster=T9 {"命令"="多个写入", "数据"={"starting address"=0, "holding register values"=[]}} ("元素"), "数据.starting address"=u16 23, "数据.holding register values"=w187) -> (w190:T9)
        n119 = Enqueue Element At Opposite End(queue=w189, element=w190) -> ()  [unwired: 2 in, 3 out]
      }
      event "R23": Mouse Down {
        n120 = event-data() -> ("CtlRef"=w195:refnum<vi>)  [unwired: 1 in, 7 out]
        n121 = Two Button Dialog(message="请确认是否更改，更改后将影响实际清洗频次" ("消息")) -> (T button?=w194:bool)  [unwired: 2 in]
        n122 = case shown="真" w194 {
          tunnel: w195 -> [_ w196]
          frame False {
          }
          frame True {
            n123 = property class="DigNum (严格)"(reference=w196) -> (reference out=w198:refnum<vi>, "Value"=w199:i16)  [unwired: 1 in, 1 out]
            n124 = call "数字键盘.vi"("OldNumber"=w199) -> ("NewNumber"=w197:sgl)
            n125 = property class="DigNum (严格)"(reference=w198, "Val(Sgnl)"=w197) -> ()  [unwired: 1 in, 2 out]
          }
        }
      }
      event "R100", "R101", "R102", "R103", "R104", "R105", "R106", "R107", "R108", "R109", "R111", "R112", "R113", "R117", "R118": Mouse Down {
        n126 = event-data() -> ("CtlRef"=w203:refnum<vi>)  [unwired: 1 in, 7 out]
        n127 = property class="DigNum (严格)"(reference=w203) -> (reference out=w201:refnum<vi>, "Value"=w202:i16)  [unwired: 1 in, 1 out]
        n128 = call "数字键盘.vi"("OldNumber"=w202) -> ("NewNumber"=w200:sgl)
        n129 = property class="DigNum (严格)"(reference=w201, "Val(Sgnl)"=w200) -> ()  [unwired: 1 in, 2 out]
      }
      event "参数设置": Value Change {
        n130 = event-data() -> ()  [unwired: 1 in, 6 out]
        n131 = property on="窗格" class="Pane"("Origin"=T1 {"Horizontal"=0, "Vertical"=628} ("原点")) -> ()  [unwired: 2 in, 2 out]
      }
      event "返回": Value Change {
        n132 = event-data() -> ()  [unwired: 1 in, 6 out]
        n133 = property on="窗格" class="Pane"("Origin"=T1 {"Horizontal"=0, "Vertical"=0} ("原点")) -> ()  [unwired: 2 in, 2 out]
      }
      event "M1-1", "V1", "M2", "V2", "V3", "V4", "V5", "V6": Value Change {
        n134 = event-data() -> ()  [unwired: 1 in, 6 out]
        n135 = Build Array("M1-1", "V1", "M2", "V2", "V3", "V4", "V5", "V6") -> (w206:bool[])
        n136 = Bundle By Name(cluster=T10 {"命令"="线圈写入", "data"={"starting address"=2400, "coil values"=[]}} ("元素"), "data.coil values"=w206) -> (w207:T10)
        n137 = Enqueue Element(queue=w217, element=w207) -> ()  [unwired: 2 in, 3 out]
      }
      event "M1-2": Value Change {
        n138 = event-data() -> ()  [unwired: 1 in, 6 out]
        n139 = Build Array("M1-2") -> (w220:bool[])
        n140 = Bundle By Name(cluster=T10 {"命令"="线圈写入", "data"={"starting address"=2413, "coil values"=[]}} ("元素"), "data.coil values"=w220) -> (w221:T10)
        n141 = Enqueue Element(queue=w219, element=w221) -> ()  [unwired: 2 in, 3 out]
      }
      event "看门狗启用": Value Change {
        n142 = event-data() -> ()  [unwired: 1 in, 6 out]
        n143 = Build Array("看门狗启用") -> (w225:bool[])
        n144 = Bundle By Name(cluster=T10 {"命令"="线圈写入", "data"={"starting address"=2801, "coil values"=[]}} ("元素"), "data.coil values"=w225) -> (w226:T10)
        n145 = Enqueue Element(queue=w224, element=w226) -> ()  [unwired: 2 in, 3 out]
      }
      event "V13NO": Value Change {
        n146 = event-data() -> ()  [unwired: 1 in, 6 out]
        n147 = Build Array("V13NO") -> (w230:bool[])
        n148 = Bundle By Name(cluster=T10 {"命令"="线圈写入", "data"={"starting address"=2414, "coil values"=[]}} ("元素"), "data.coil values"=w230) -> (w231:T10)
        n149 = Enqueue Element(queue=w229, element=w231) -> ()  [unwired: 2 in, 3 out]
      }
      event "V13NC": Value Change {
        n150 = event-data() -> ()  [unwired: 1 in, 6 out]
        n151 = Build Array("V13NC") -> (w235:bool[])
        n152 = Bundle By Name(cluster=T10 {"命令"="线圈写入", "data"={"starting address"=2415, "coil values"=[]}} ("元素"), "data.coil values"=w235) -> (w236:T10)
        n153 = Enqueue Element(queue=w234, element=w236) -> ()  [unwired: 2 in, 3 out]
      }
      event "V14NO": Value Change {
        n154 = event-data() -> ()  [unwired: 1 in, 6 out]
        n155 = Build Array("V14NO") -> (w240:bool[])
        n156 = Bundle By Name(cluster=T10 {"命令"="线圈写入", "data"={"starting address"=2408, "coil values"=[]}} ("元素"), "data.coil values"=w240) -> (w241:T10)
        n157 = Enqueue Element(queue=w239, element=w241) -> ()  [unwired: 2 in, 3 out]
      }
      event "V14NC": Value Change {
        n158 = event-data() -> ()  [unwired: 1 in, 6 out]
        n159 = Build Array("V14NC") -> (w245:bool[])
        n160 = Bundle By Name(cluster=T10 {"命令"="线圈写入", "data"={"starting address"=2409, "coil values"=[]}} ("元素"), "data.coil values"=w245) -> (w246:T10)
        n161 = Enqueue Element(queue=w244, element=w246) -> ()  [unwired: 2 in, 3 out]
      }
    }
  }
  n162 = Enqueue Element(queue=w12, element=cluster{"命令":string, "数据":variant} {"命令"="init", "数据"=variant} ("元素"), error in (no error)=w11) -> (queue out=w7:refnum<queue>, error out=w9:errorcluster)  [unwired: 1 in, 1 out]
  n163 = while {
    tunnel: w7 -> [w252]
    tunnel: w9 -> [w251]
    shift-right: [w255] -> w4
    shift-left: refnum<class "MB_Master.lvclass"> refnum ("MB session in") -> [w254]
    tunnel: errorcluster {"status"=FALSE, "code"=0, "source"=""} ("error out") -> [w253]
    tunnel: [w250] -> w5
    stop <- FALSE stop-if-true
    n164 = case shown="无错误" w253 {
      selector: w253 -> [w260 w442]
      tunnel: [w263 w441] -> w255
      tunnel: w254 -> [w262 w443]
      tunnel: [w261 w439] -> w250
      tunnel: w252 -> [w258 w438]
      tunnel: w251 -> [w257 _]
      frame No Error {
        n165 = Dequeue Element(queue=w258, error in (no error)=w257) -> (element=w256:cluster{"命令":string, "数据":variant})  [unwired: 1 in, 3 out]
        n166 = Unbundle By Name(w256) -> ("命令"=w259:string)
        n167 = case shown="\"读状态\"" w259 {
          tunnel: [w265 w278 w301 w382 w394 w404 w414 w424] -> w263
          tunnel: w262 -> [w265 w280 w352 w387 w397 w407 w417 w427]
          tunnel: [w264 w279 w299 w381 w395 w405 w415 w418] -> w261
          tunnel: w260 -> [w264 w282 w355 w386 w396 w406 w416 w425]
          tunnel: w256 -> [_ _ _ _ w393 w403 w413 _]
          frame "idle", Default {
          }
          frame "init" {
            w270 = refnum<visa-resource-name> "COM3" ("VISA resource name")
            n168 = call-dynamic "Close Session.vi"("error in (no error)"=w282, "MB session in"=w280) -> ("error out"=w281:errorcluster)  [unwired: 9 in]
            n169 = call <vilib>:"Clear Errors.vi"("error in (no error)"=w281) -> ("error out"=w268:errorcluster)  [unwired: 5 in, 1 out]
            n170 = call-poly "VISA Configure Serial Port"("VISA resource name"=w270, "baud rate (9600)"=u32 115200, "error in (no error)"=w268) -> ("VISA resource name out"=w272:refnum<visa-resource-name>, "error out"=w274:errorcluster)  [unwired: 11 in]
            n171 = VISA Write(VISA resource name=w272, write buffer="\u0002004701R04047560A5B\u0003" ("写入缓冲区"), error in (no error)=w274) -> (VISA resource name out=w271:refnum<visa-resource-name>, error out=w273:errorcluster)  [unwired: 1 out]
            n172 = VISA Close(VISA resource name=w271, error in (no error)=w273) -> (error out=w267:errorcluster)
            n173 = call <vilib>:"Open Serial Session.vi"("Mode (RTU)"=enum16{"RTU", "ASCII"}."RTU", "Error in"=w267, "Slave ID"=u8 10, "Serial Config"=T13 {"baud rate (bps)"=115200, "stop bits"=10, "parity"=0, "flow control"=0, "timeout"=500, "retries"=1}, "VISA Resource"=w270) -> ("Error out"=w279:errorcluster, "MB_Serial session"=w278:refnum<class "MB_Master_Serial.lvclass">)  [unwired: 5 in]
            n174 = Unbundle By Name(w279) -> ("status"=w283:bool)
            n175 = call "对话框信息"("Enable"=w283) -> ()  [unwired: 9 in, 2 out]
          }
          frame "读状态" {
            n176 = call <vilib>:"Read Holding Registers.vi"("error in (no error)"=w355, "quantity"=u16 44 ("number of holding registers"), "starting address"=u16 0, "MB session in"=w352) -> ("error out"=w350:errorcluster, "Registers"=w288:u16[], "MB session out"=w351:refnum<class "MB_Master.lvclass">)  [unwired: 5 in]
            n177 = Array Subset(array=w288, index=36 ("索引"), length=8 ("长度")) -> (w291:u16[])
            n178 = Array Subset(array=w288, index=27 ("索引")) -> (w320:u16[])  [unwired: 1 in]
            n179 = Array To Cluster(array=w288) -> (cluster=w294:T17)
            n180 = call "浮点CDAB转换.vi"("数组"=w291) -> ("数组 2"=w290:sgl[])  [unwired: 10 in]
            n181 = global write "采配水全局变量.vi" "状态"(w294) -> ()
            n182 = Index Array(array=w288, index=35 ("索引")) -> (element=w286:u16)
            n183 = Insert Into Array(array=w290, index=0 ("索引"), new element=w286) -> (w285:sgl[])
            n184 = call <vilib>:"Read Holding Registers.vi"("error in (no error)"=w350, "quantity"=u16 6 ("number of holding registers"), "starting address"=u16 3840, "MB session in"=w351) -> ("error out"=w346:errorcluster, "Registers"=w323:u16[], "MB session out"=w347:refnum<class "MB_Master.lvclass">)  [unwired: 5 in]
            n185 = Array To Cluster(array=w285) -> (cluster=w284:T18)
            n186 = global write "采配水全局变量.vi" "空调状态"(w284) -> ()
            n187 = To Word Integer(number=w323) -> (16bit integer=w322:i16[])
            n188 = call "FATEK_HexToString.vi"("数组"=w320) -> ("STRING"=w319:string[])  [unwired: 10 in]
            n189 = Array To Cluster(array=w323) -> (cluster=w363:T19)
            n190 = global write "采配水全局变量.vi" "AD"(w363) -> ()
            n191 = formula code="float AD0,AD1,AD2,AD3,AD4,AD5,AD6;\nAD0 = IN[0]*140/6553-75;\nAD1 = IN[1]/65.53-25;\nAD2 = IN[2]*30/8191;\nAD3 = IN[3]*30/8191;\nAD4 = IN[4]*30/8191;\nAD5 = IN[5]*30/8191;"("IN"=w322) -> ("AD0"=w361:dbl, "AD1"=w360:dbl, "AD2"=w359:dbl, "AD3"=w358:dbl, "AD4"=w357:dbl, "AD5"=w356:dbl)
            n192 = Index Array(array=w319) -> (element=→"采配水版本号":string)  [unwired: 1 in]
            n193 = call <vilib>:"Read Coils.vi"("error in (no error)"=w346, "quantity"=u16 32 ("number of coils"), "starting address"=u16 0, "MB session in"=w347) -> ("error out"=w342:errorcluster, "Coils"=w327:bool[], "MB session out"=w343:refnum<class "MB_Master.lvclass">)  [unwired: 5 in]
            n194 = global write "采配水全局变量.vi" "输出状态"(w327) -> ()
            n195 = Bundle(w361, w360, w359, w358, w357, w356) -> (w362:cluster{dbl, dbl, dbl, dbl, dbl, dbl})  [unwired: 1 in]
            n196 = Index Array(array=w327, index #7=13 ("索引")) -> (element #1=w317:bool, element #2=w316:bool, element #3=w315:bool, element #4=w314:bool, element #5=w313:bool, element #6=w312:bool, element #7=w310:bool, element #8=w309:bool, element #11=w308:bool, element #12=w307:bool, element #14=w303:bool)  [unwired: 13 in, 3 out]
            n197 = global write "采配水全局变量.vi" "转换值"(w362) -> ()
            n198 = call <vilib>:"Read Coils.vi"("error in (no error)"=w342, "quantity"=u16 16 ("number of coils"), "starting address"=u16 1000, "MB session in"=w343) -> ("error out"=w338:errorcluster, "Coils"=w334:bool[], "MB session out"=w339:refnum<class "MB_Master.lvclass">)  [unwired: 5 in]
            n199 = local write "V1"(w317) -> ()
            n200 = local write "V2"(w316) -> ()
            n201 = local write "V3"(w315) -> ()
            n202 = local write "V4"(w314) -> ()
            n203 = local write "V5"(w313) -> ()
            n204 = local write "V6"(w312) -> ()
            n205 = local write "M1-1"(w308) -> ()
            n206 = local write "M1-2"(w307) -> ()
            n207 = local write "M2"(w303) -> ()
            n208 = global write "采配水全局变量.vi" "输入状态"(w334) -> ()
            n209 = Index Array(array=w334) -> (element #1=→"X0":bool, element #2=→"X1":bool, element #3=→"X2":bool, element #4=→"X3":bool, element #5=→"X4":bool, element #6=→"X5":bool, element #7=→"X6":bool, element #8=→"X7":bool, element #9=→"X8":bool, element #10=→"X9":bool, element #11=→"X10":bool, element #12=→"X11":bool)  [unwired: 12 in]
            n210 = local write "V13NO"(w310) -> ()
            n211 = local write "V13NC"(w309) -> ()
            n212 = call <vilib>:"Read Coils.vi"("error in (no error)"=w338, "quantity"=u16 16 ("number of coils"), "starting address"=u16 2500, "MB session in"=w339) -> ("error out"=w300:errorcluster, "Coils"=w335:bool[], "MB session out"=w302:refnum<class "MB_Master.lvclass">)  [unwired: 5 in]
            n213 = global write "采配水全局变量.vi" "报警簇"(w335) -> ()
            n214 = call <vilib>:"Read Coils.vi"("error in (no error)"=w300, "quantity"=u16 1 ("starting address"), "starting address"=u16 2801, "MB session in"=w302) -> ("error out"=w299:errorcluster, "Coils"=w296:bool[], "MB session out"=w301:refnum<class "MB_Master.lvclass">)  [unwired: 5 in]
            n215 = Index Array(array=w296) -> (element=w295:bool)  [unwired: 1 in]
            n216 = local write "看门狗启用"(w295) -> ()
          }
          frame "读参数" {
            n217 = call <vilib>:"Read Holding Registers.vi"("error in (no error)"=w386, "quantity"=u16 20 ("number of holding registers"), "starting address"=u16 100, "MB session in"=w387) -> ("error out"=w381:errorcluster, "Registers"=w383:u16[], "MB session out"=w382:refnum<class "MB_Master.lvclass">)  [unwired: 5 in]
            n218 = Array To Cluster(array=w383) -> (cluster=w370:T20)
            n219 = global write "采配水全局变量.vi" "参数设置"(w370) -> ()
            n220 = Unbundle(w370) -> ("Registers[0]"=→"R100":u16, "Registers[1]"=→"R101":u16, "Registers[2]"=→"R102":u16, "Registers[3]"=→"R103":u16, "Registers[4]"=→"R104":u16, "Registers[5]"=→"R105":u16, "Registers[6]"=→"R106":u16, "Registers[7]"=→"R107":u16, "Registers[8]"=→"R108":u16, "Registers[9]"=→"R109":u16, "Registers[10]"=w369:u16, "Registers[11]"=→"R111":u16, "Registers[12]"=→"R112":u16, "Registers[13]"=→"R113":u16, "Registers[16]"=w365:u16, "Registers[18]"=→"R118":u16)  [unwired: 4 out]
            n221 = local write "R116"(w365) -> ()
            n222 = local write "潜水泵工作模式"(w369) -> ()
          }
          frame "多个写入" {
            n223 = Unbundle By Name(w393) -> ("数据"=w392:variant)
            n224 = Variant To Data(type=T14 {"starting address"=0, "holding register values"=[]}, Variant=w392) -> (data=w390:T14)  [unwired: 1 in, 1 out]
            n225 = Unbundle By Name(w390) -> ("starting address"=w389:u16, "holding register values"=w388:u16[])
            n226 = call <vilib>:"Write Multiple Registers.vi"("error in (no error)"=w396, "values"=w388, "starting address"=w389, "MB session in"=w397) -> ("error out"=w395:errorcluster, "MB session out"=w394:refnum<class "MB_Master.lvclass">)  [unwired: 6 in]
          }
          frame "单个写入" {
            n227 = Unbundle By Name(w403) -> ("数据"=w402:variant)
            n228 = Variant To Data(type=T15 {"starting address"=0, "holding register value"=0}, Variant=w402) -> (data=w400:T15)  [unwired: 1 in, 1 out]
            n229 = Unbundle By Name(w400) -> ("starting address"=w399:u16, "holding register value"=w398:u16)
            n230 = call <vilib>:"Write Single Register.vi"("error in (no error)"=w406, "value"=w398, "address"=w399, "MB session in"=w407) -> ("error out"=w405:errorcluster, "MB session out"=w404:refnum<class "MB_Master.lvclass">)  [unwired: 6 in]
          }
          frame "线圈写入" {
            n231 = Unbundle By Name(w413) -> ("数据"=w412:variant)
            n232 = Variant To Data(type=T16 {"starting address"=0, "coil values"=[]}, Variant=w412) -> (data=w410:T16)  [unwired: 1 in, 1 out]
            n233 = Unbundle By Name(w410) -> ("starting address"=w409:u16, "coil values"=w408:bool[])
            n234 = call <vilib>:"Write Multiple Coils.vi"("error in (no error)"=w416, "values"=w408, "starting address"=w409, "MB session in"=w417) -> ("error out"=w415:errorcluster, "MB session out"=w414:refnum<class "MB_Master.lvclass">)  [unwired: 6 in]
          }
          frame "shutdown" {
            n235 = call <vilib>:"Write Single Register.vi"("error in (no error)"=w425, "value"=u16 0, "address"=u16 4047, "MB session in"=w427) -> ("error out"=w426:errorcluster, "MB session out"=w424:refnum<class "MB_Master.lvclass">)  [unwired: 6 in]
            n236 = call "文件对话框"("start path"=path "D:/SRC") -> ("selected path"=w421:path, "cancelled"=w419:bool)  [unwired: 11 in, 2 out]
            n237 = call-dynamic "Close Session.vi"("error in (no error)"=w426, "MB session in"=w424) -> ("error out"=w418:errorcluster)  [unwired: 9 in]
            n238 = case shown="假" w419 {
              tunnel: w421 -> [w432 _]
              tunnel: w418 -> [_ _]
              frame False {
                n239 = Path To String(path=w432) -> (string=w429:string)
                n240 = Format Into String(format string="  - \"%s\"" ("格式字符串"), initial string="\"C:\\Program Files\\Fatek\\WinProladder\\WProlad.exe\"" ("command line"), w429) -> (resulting string=w430:string)  [unwired: 1 in, 1 out]
                n241 = call <vilib>:"System Exec.vi"("command line"=w430) -> ("error out"=w433:errorcluster)  [unwired: 7 in, 3 out]
                n242 = case shown="错误" w433 {
                  tunnel: w429 -> [_ w436]
                  frame No Error {
                  }
                  frame Error {
                    n243 = Format Into String(format string="  - \"%s\"" ("格式字符串"), initial string="\"C:\\Program Files (x86)\\Fatek\\WinProladder\\WProlad.exe\"" ("command line"), w436) -> (resulting string=w434:string)  [unwired: 1 in, 1 out]
                    n244 = call <vilib>:"System Exec.vi"("command line"=w434) -> ()  [unwired: 7 in, 4 out]
                  }
                }
              }
              frame True {
              }
            }
          }
        }
      }
      frame Error {
        n245 = Unbundle By Name(w442) -> ("code"=w444:i32)
        n246 = case shown="-1073807343" w444 {
          tunnel: w443 -> [w446 w450]
          tunnel: w442 -> [w445 w452]
          tunnel: [w445 w451] -> w440
          tunnel: [w446 w450] -> w441
          tunnel: w438 -> [_ w449]
          frame Default {
          }
          frame -1073807343 {
            n247 = Flush Queue(queue=w449) -> (queue out=w448:refnum<queue>)  [unwired: 1 in, 2 out]
            n248 = call-dynamic "Close Session.vi"("error in (no error)"=w452, "MB session in"=w450) -> ("error out"=w451:errorcluster)  [unwired: 9 in]
            n249 = disable-structure shown="禁用" {
              disable-tunnel: w448 -> [w453 _]
              frame Disabled {
                n250 = Enqueue Element At Opposite End(queue=w453, element=cluster{"命令":string, "数据":variant} {"命令"="init", "数据"=variant} ("元素")) -> ()  [unwired: 2 in, 3 out]
              }
              frame Enabled {
              }
            }
            n251 = Wait (ms)(milliseconds to wait=u32 2000 ("等待时间（毫秒）")) -> ()  [unwired: 1 out]
          }
        }
        n252 = call <vilib>:"Clear Errors.vi"("error in (no error)"=w440) -> ("error out"=w439:errorcluster)  [unwired: 5 in, 1 out]
      }
    }
    n253 = Unbundle By Name(w250) -> ("status"=→"通讯故障":bool)
  }
  n254 = property on="多列列表框" class="MCListbox (严格)"("ItemNames"=string[][] [["待机"], ["初始化"], ["外部管路润洗"], ["内部管路润洗"], ["采样"], ["沉淀"], ["配水"], ["外部管路反冲洗"], ["内部管路反冲洗"], ["采样池储水"], ["结束"]] ("项名")) -> ()  [unwired: 2 in, 2 out]
  n255 = call-dynamic "Close Session.vi"("error in (no error)"=w5, "MB session in"=w4) -> ()  [unwired: 9 in, 1 out]
